vi "LoadFiles.vi"(5 "FileListIn in":string[](array[string]), 6 "Cluster":T2, 7 "FileList":string[](array[string]), 8 "Downsample":i32, 9 "DEMP Folder":path, 10 "MessageBox":refnum<vi>, 11 "FileDictionary":refnum<k24>) -> (0 "FileListIn out":string[](array[string]), 1 "Channels":string[](array[string]), 2 "Keys":string[](array[string]), 3 "DataPile":T1(array[cluster]), 4 "dt":dbl)   [LabVIEW 2024]
uses:
  E:/CodeProjects/DEMPViewer/ClassLibrary1.dll
  ClassLibrary1.dll
  <vilib>/regexp/Match Regular Expression.xnode
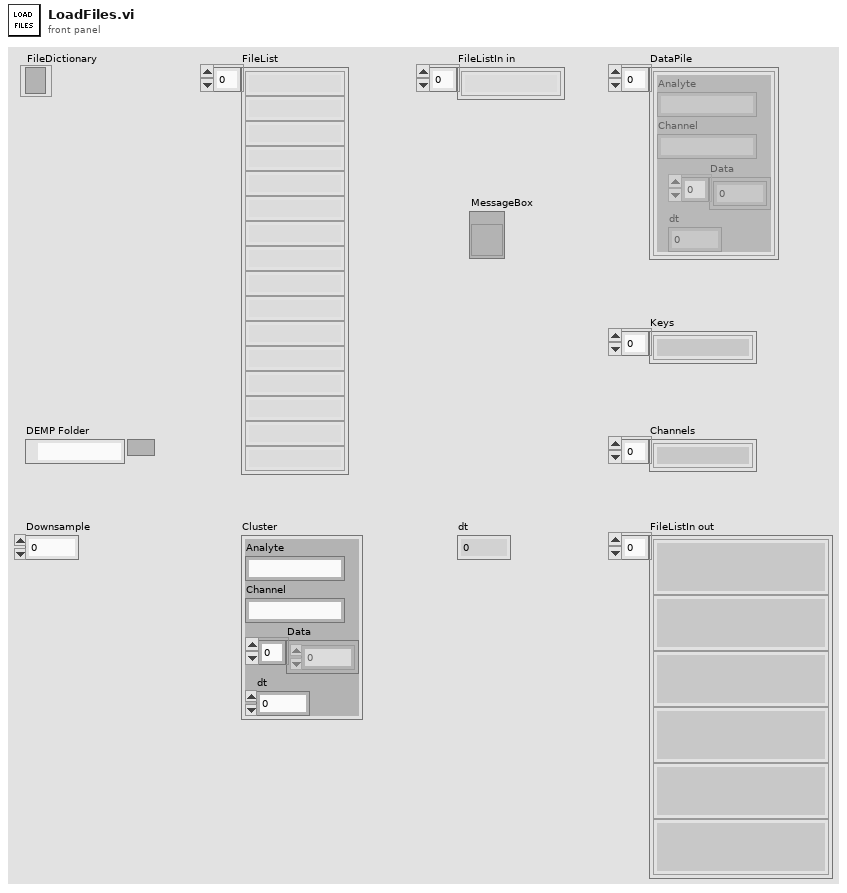
[diagram p1: front panel]
types:
  T1 = cluster{"Analyte":string, "Channel":string, "Data":dbl[], "dt":dbl}[]
  T2 = cluster{"Analyte":string, "Channel":string, "Data":dbl[], "dt":dbl}
  T3 = enum16{"open", "open or create", "create or replace", "create", "open (read-only)"}
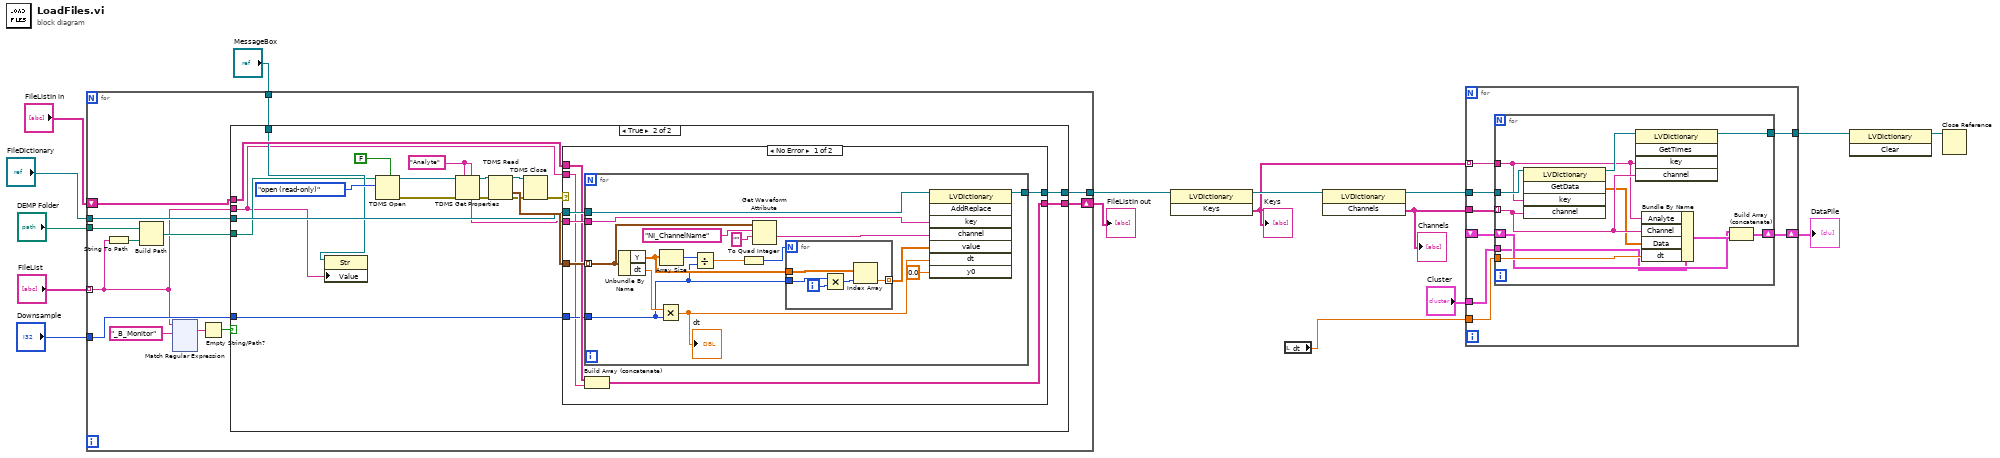
[diagram p0: block diagram]
diagram:
  n1 = for {
    tunnel: "FileList" -> [w19] mode=indexing
    tunnel: "DEMP Folder" -> [w29]
    tunnel: "FileDictionary" -> [w24]
    tunnel: [w23] -> w13
    shift-right: [w22] -> w3
    shift-left: "FileListIn in" -> [w21]
    tunnel: "Downsample" -> [w20]
    tunnel: "MessageBox" -> [w18]
    n2 = String To Path(string=w19) -> (path=w30:path)
    n3 = Build Path(base path=w29, name or relative path=w30) -> (appended path=w28:path)
    n4 = xnode "Match Regular Expression"("input string"=w19, "regular expression"="_B_Monitor") -> ("whole match"=w26:string)  [unwired: 4 in, 4 out]
    n5 = Empty String/Path?(string/path=w26) -> (empty?=w25:bool)
    n6 = case shown="True" w25 {
      tunnel: w28 -> [_ w34]
      tunnel: w24 -> [w32 w45]
      tunnel: [w32 w43] -> w23
      tunnel: [w31 w42] -> w22
      tunnel: w21 -> [w31 w41]
      tunnel: w20 -> [_ w40]
      tunnel: w19 -> [_ w33]
      tunnel: w18 -> [_ w35]
      frame False {
      }
      frame True {
        w47 = "Analyte" ("property name")
        n7 = property on="Property Node" class="Str"(reference=w35, "Value"=w33) -> ()  [unwired: 1 in, 2 out]
        n8 = TDMS Open(5:FALSE ("create index file? (T)"), 10:T3."open (read-only)" ("operation (0:open)"), 11:w34) -> (0:w39:errorcluster, 3:w49:refnum<k34>)  [unwired: 4 in]
        n9 = TDMS Get Properties(5:w47, 7:w47, 8:w39, 11:w49) -> (0:w38:errorcluster, 3:w48:refnum<k34>, 4:w44:string)  [unwired: 2 in, 3 out]
        n10 = TDMS Read(0:w48, 11:w38) -> (4:w50:refnum<k34>, 10:w46:waveform(dbl)[], 15:w37:errorcluster)  [unwired: 6 in, 3 out]
        n11 = TDMS Close(8:w37, 11:w50) -> (0:w36:errorcluster)  [unwired: 1 out]
        n12 = case shown="No Error" w36 {
          tunnel: w46 -> [w60 _]
          tunnel: w45 -> [w59 w83]
          tunnel: w44 -> [w58 _]
          tunnel: [w57 w83] -> w43
          tunnel: [w56 w82] -> w42
          tunnel: w41 -> [w55 w82]
          tunnel: w40 -> [w54 _]
          tunnel: w33 -> [w53 _]
          frame No Error {
            n13 = for {
              tunnel: w60 -> [w70] mode=indexing
              tunnel: w59 -> [w75]
              tunnel: w58 -> [w74]
              tunnel: [w73] -> w57
              tunnel: w54 -> [w61]
              n14 = Unbundle By Name(w70) -> ("Y"=w67:dbl[], "dt"=w76:dbl)
              n15 = Multiply(x=w76, y=w61) -> (x*y=w62:dbl)
              "dt" <- w62
              n16 = Array Size(array=w67) -> (size(s)=w66:i32)
              n17 = Divide(x=w66, y=w61) -> (x/y=w65:dbl)
              n18 = To Quad Integer(1:w65) -> (0:w64:i64)
              n19 = Get Waveform Attribute(5:"", 6:"NI_ChannelName" ("name"), 7:w70) -> (1:w69:string)  [unwired: 1 in, 3 out]
              n20 = for {
                N: w64 -> [_]
                tunnel: w67 -> [w81]
                tunnel: w61 -> [w78]
                tunnel: [w77] -> w63 mode=indexing
                i -> [w80]
                n21 = Multiply(x=w78, y=w80) -> (x*y=w79:i32)
                n22 = Index Array(array=w81, index=w79) -> (element=w77:dbl)
              }
              n23 = invoke class="LVDictionary" method="AddReplace"(reference=w75, "key"=w74, "channel"=w69, "value"=w63, "dt"=w62, "y0"=0.0) -> (reference out=w73:refnum<k24>)  [unwired: 2 in, 7 out]
            }
            n24 = Build Array (concatenate)(w55, w53) -> (w56:string[])
          }
          frame Error {
          }
        }
      }
    }
  }
  "FileListIn out" <- w3
  n25 = invoke class="LVDictionary" method="Keys"(reference=w13) -> (reference out=w12:refnum<k24>, "Keys"=w10:string[])  [unwired: 2 in, 1 out]
  "Keys" <- w10
  n26 = local read "dt"() -> (w2:dbl)
  n27 = invoke class="LVDictionary" method="Channels"(reference=w12) -> (reference out=w11:refnum<k24>, "Channels"=w8:string[])  [unwired: 2 in, 1 out]
  "Channels" <- w8
  n28 = for {
    tunnel: w11 -> [w208]
    tunnel: w10 -> [w205] mode=indexing
    tunnel: w8 -> [w207]
    tunnel: "Cluster" -> [w202]
    tunnel: w2 -> [w206]
    shift-right: [w204] -> w7
    shift-left: _ -> [w203]
    tunnel: [w201] -> w6
    n29 = for {
      tunnel: w208 -> [w219]
      tunnel: w207 -> [w217] mode=indexing
      tunnel: w206 -> [w215]
      tunnel: w205 -> [w214]
      shift-right: [w212] -> w204
      shift-left: w203 -> [w211]
      tunnel: w202 -> [w210]
      tunnel: [w209] -> w201
      n30 = invoke class="LVDictionary" method="GetData"(reference=w219, "key"=w214, "channel"=w217) -> (reference out=w218:refnum<k24>, "GetData"=w216:dbl[])  [unwired: 2 in, 3 out]
      n31 = invoke class="LVDictionary" method="GetTimes"(reference=w218, "key"=w214, "channel"=w217) -> (reference out=w209:refnum<k24>)  [unwired: 2 in, 4 out]
      n32 = Bundle By Name(cluster=w210, "Analyte"=w214, "Channel"=w217, "Data"=w216, "dt"=w215) -> (w213:T2)
      n33 = Build Array (concatenate)(w211, w213) -> (w212:T1)
    }
  }
  "DataPile" <- w7
  n34 = invoke class="LVDictionary" method="Clear"(reference=w6) -> (reference out=w5:refnum<k24>)  [unwired: 2 in, 2 out]
  n35 = Close Reference(reference=w5) -> ()  [unwired: 1 in, 1 out]
